vi "dvp Vi Get Ae Operation.vi"(10 "pAeOperation":u32(ring) items=["AE_OP_OFF", "AE_OP_ONCE", "AE_OP_CONTINUOUS"], 11 "handle":u32) -> (2 "pAeOperation out":u32(ring) items=["AE_OP_OFF", "AE_OP_ONCE", "AE_OP_CONTINUOUS"], 3 "function return":u32(ring))   [LabVIEW 2018, in "LabViewDVPCamera.lvlib"]
doc: "LabviewDvp2Api dvpStatus dvpViGetAeOperation(dvpHandle handle, dvpAeOperation *pAeOperation);"
uses:
  LabViewDVPCamera.lvlib
  LabViewDVPCamera/LabViewDVPCamera.dll
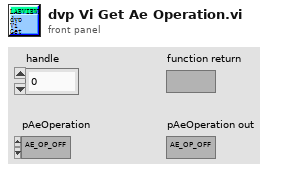
[diagram p1: front panel]
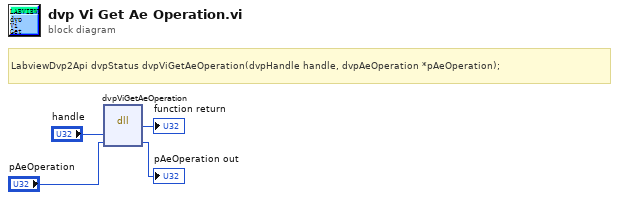
[diagram p0: block diagram]
diagram:
  # "LabviewDvp2Api dvpStatus dvpViGetAeOperation(dvpHandle handle, dvpAeOperation *pAeOperation);"
  n1 = dll-call lib="C:/Program Files (x86)/DVP2 Labview cn 64/Sample/LabViewDVPCamera/LabViewDVPCamera.*" fn="dvpViGetAeOperation"("handle"="handle", "pAeOperation"="pAeOperation") -> (→"function return":u32, "pAeOperation"=→"pAeOperation out":u32)  [unwired: 4 in, 2 out]
